vi "play-AFM-CS-imaging_v3.vi"() -> ()   [LabVIEW 2017]
uses:
  controls/boolean_info.ctl
  controls/z-axis-params_v3.ctl
  controls/TF-params.ctl
  <userlib>/_matio/level5/Public/MAT-File Data Types.ctl
  <vilib>/userdefined/High Color/nirio_resource_hc.ctl
  controls/expMetaData.ctl
  <vilib>/Utility/file.llb/Read Delimited Spreadsheet (DBL).vi
  <vilib>/FPGAPlugInAG/cRIO-9082/niLvFpga_Open_cRIO-9082.vi
  <vilib>/rvi/interface/common/dynamic/niFpgaDynamicAddResources.vi
  <vilib>/FPGAPlugInAG/Dynamic/niLvFpga_Reset_Dynamic.vi
  <vilib>/rvi/interface/common/niFpgaWaitOnOcc.vi
  <vilib>/Utility/error.llb/Error Cluster From Error Code.vi
  <vilib>/rvi/errors/niLvFpgaAdjustHostInterfaceError.vi
  <vilib>/FPGAPlugInAG/Dynamic/niLvFpga_Run_Dynamic.vi
  fpga_interface_lib/acquire_FXP_16-5_FIFO_2.vi
  <vilib>/Utility/file.llb/Write Delimited Spreadsheet (DBL).vi
  <vilib>/FPGAPlugInAG/Dynamic/niLvFpga_Close_Dynamic.vi
  <userlib>/_matio/level5/Public/Write/Append Data Element.llb/Append Data Element (Anything).vi
  <vilib>/rvi/interface/nirviOpenFPGA/nirviOpenFPGA.xnode
  FPGA Bitfiles/afmimagingcontro_FPGATargetSPARTA_cs-scanningv3.lvbitx
  <vilib>/rvi/interface/nirviMethod/nirviMethod.xnode
  <vilib>/rvi/interface/nirviReadWriteControl/nirviReadWriteControl.xnode
  <vilib>/rvi/interface/nirviCloseFPGA/nirviCloseFPGA.xnode
  <vilib>/FPGAPlugInAG/Dynamic/niLvFpga_ConfigureFifo_Dynamic.vi
  <vilib>/rvi/errors/niLvFpgaMergeErrorWithErrorCode.vi
  <vilib>/rvi/interface/Simulation/niFpgaSimulationCallBeginRW.vi
  NiFpgaLv.dll
  <userlib>/_matio/level5.lvlib
  fpga_interface_lib/fpga_interface.lvlib
panel:
  in  "do-Dz":bool
  in  "TF-params":T1={"TF-order"=2, "Num"=[1.0237086, -2.0434425, 1.0225973, 0.0, 0.0, 0.0, 0.0, 0.0, 0.0], "Den"=[1.0, -1.9961116, 0.998975, 0.0, 0.0, 0.0, 0.0, 0.0, 0.0]}
  in  "input-data-path":path
  out "boolean \nindicators":T2
  out "CS Time":dbl
  out "Current Case":i16
  out "state times":dbl[](array[numeric])
  out "entity-index":i16
  in  "Tab Control":T3(tab)
  in  "init Z up":sgl step=0.5
  in  "trigger-0":bool
  in  "numEntities":i16
  out "output-data-path":path
  out "output-meta-data-path":path
  in  "note-blob":string
  in  "overwrite":bool
  in  "TsTicks":u32=1600
  in  "Ki-xy":sgl=0.005
  in  "collect all":bool=TRUE
  in  "z_axis_params":T4={"TOL"=0.01, "ramp_rate"=-0.005, "z_u_max"=6.0, "setpoint"=0.0, "Ki"=0.04, "Z_error_threshold"=0.05, "Z_settled_samples_threshold "=500, "zup_rate"=0.1, "uz_safe"=0.60009765625, "Kiz_down"=0.04, "max_Z_settle_samples"=2500} {"uz_safe" format="%#_13g"; "Z_error_threshold" format="%#_13g"; "ramp_rate" format="%#_4g"; "TOL" format="%#_13g"}
  in  "ramp_down":bool
  in  "xy settled-samples\n threshold":i16=200
  in  "xy error-threshold":sgl=0.1
  out "number-settled-samples-x":i16
  out "number-settled-samples-y":i16
  out "case-selected":i16
  out "number-settled-samples-Z":i16
  out "size(s)":i32
  out "nsamps":i32
  out "y iter":i32
  out "size(s) 2":i32[](array[numeric])
  out "Array":i32[][](array[numeric])
  out "error out 2":errorcluster
  out "z-control":dbl[](graph)
  out "x-axis":dbl[](graph)
  out "z-error":dbl[](graph)
  out "y-axis":dbl[](graph)
  in  "STOP":bool
  # "- If collect all = fasle and collect move = false,\nwe only collect measurement data.\n- If collect all = false, and collect move = true,\nwe collect measurement and move data.\n- If collect all = true, we collect everything."
  # "move"
  # "lower"
  # "z-settle"
  # "scan"
  # "tip-up"
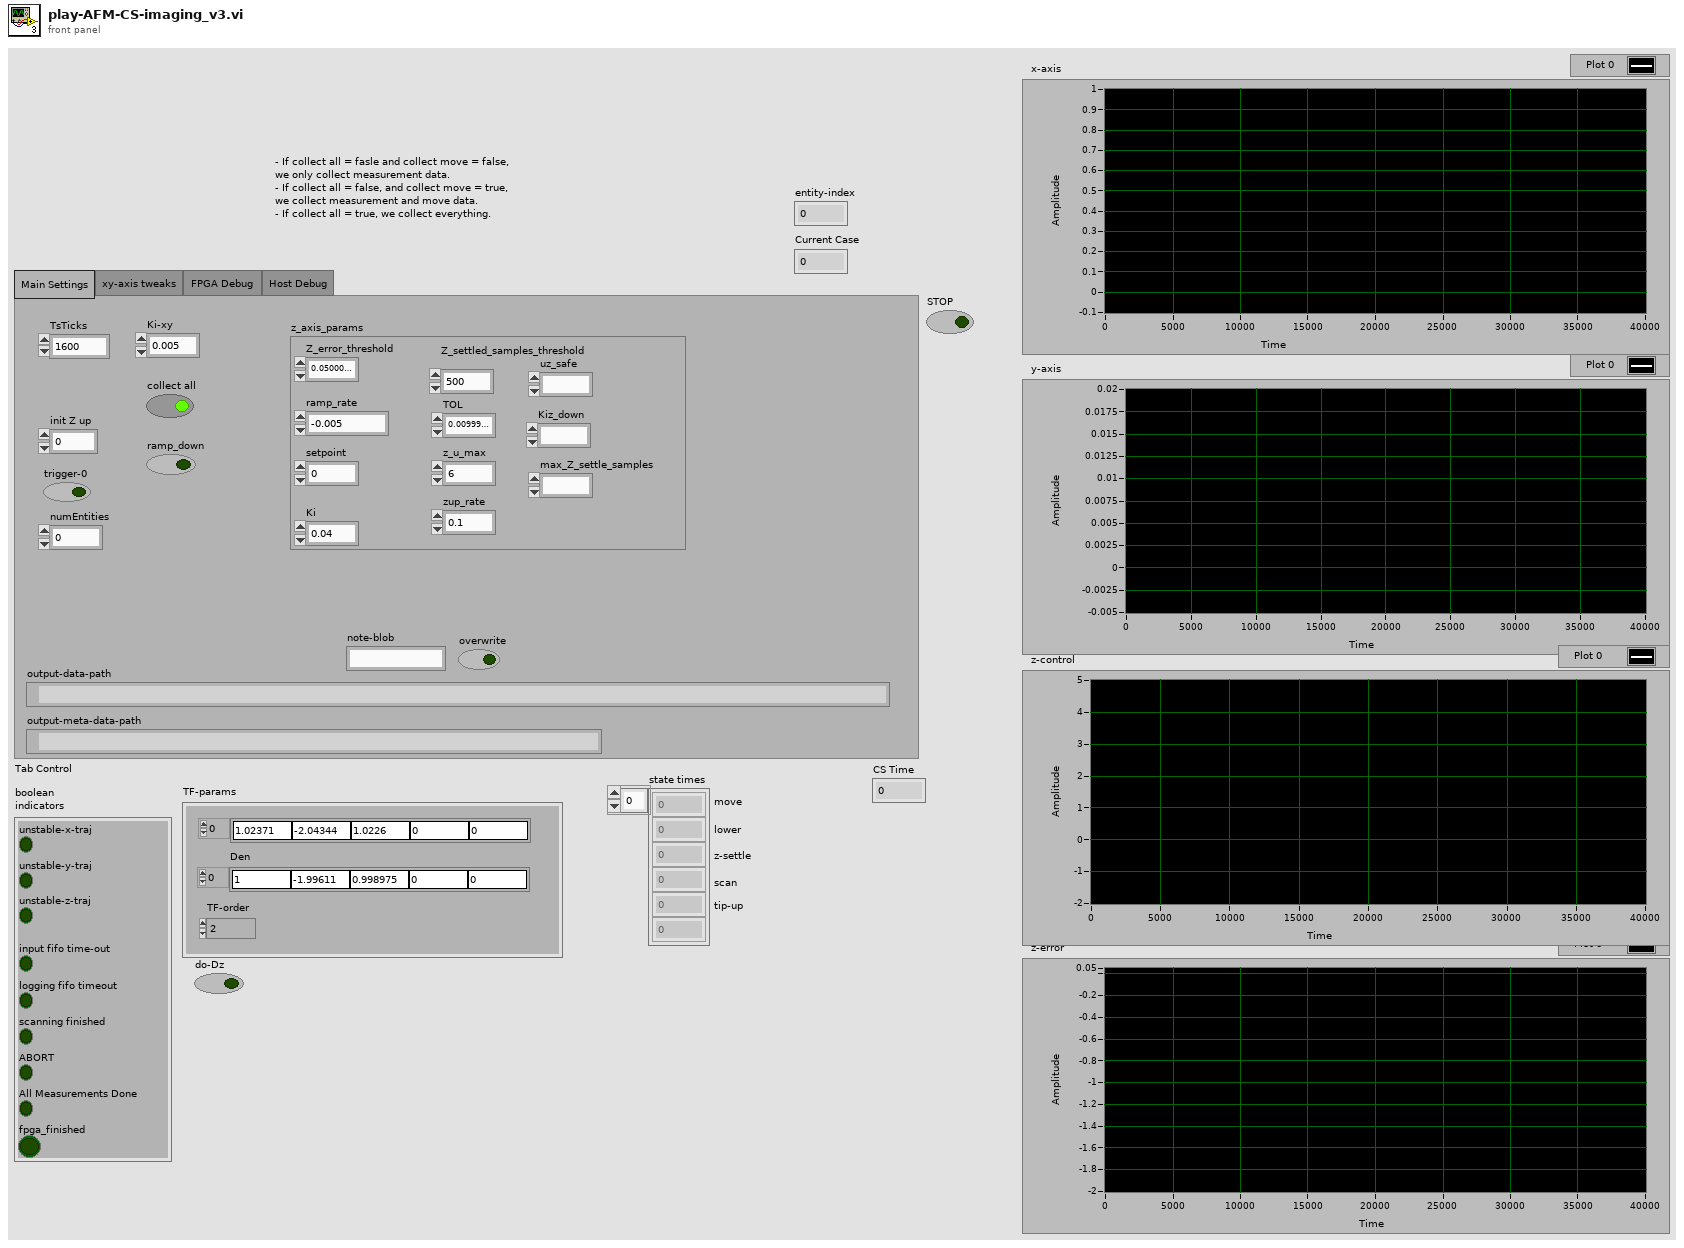
[diagram p1: front panel]
types:
  T1 = typedef "TF-params.ctl" = cluster{"TF-order":i16, "Num":sgl[], "Den":sgl[]}
  T2 = typedef "boolean_info.ctl" = cluster{"unstable-z-traj":bool, "input fifo time-out":bool, "logging fifo timeout":bool, "scanning finished":bool, "unstable-x-traj":bool, "unstable-y-traj":bool, "ABORT":bool, "All Measurements Done":bool, "fpga_finished":bool}
  T3 = enum32{"Main Settings", "xy-axis tweaks", "FPGA Debug ", "Host Debug"}
  T4 = typedef "z-axis-params_v3.ctl" = cluster{"TOL":sgl, "ramp_rate":sgl, "z_u_max":sgl, "setpoint":sgl, "Ki":sgl, "Z_error_threshold":sgl, "Z_settled_samples_threshold ":i16, "zup_rate":sgl, "uz_safe":fxp<+/-,16,5>, "Kiz_down":sgl, "max_Z_settle_samples":i16}
  T5 = typedef "level5.lvlib/MAT-File Data Types.ctl" = enum32{"_invalid", "miINT8", "miUINT8", "miINT16", "miUINT16", "miINT32", "miUINT32", "miSINGLE", "_reserved_1", "miDOUBLE", "_reserved_2", "_reserved_3", "miINT64", "miUINT64", "miMATRIX", "miCOMPRESSED", "miUTF8", "miUTF16", "miUTF32"}
  T6 = typedef "nirio_resource_hc.ctl" = tag
  T7 = cluster{"unstable-z-traj":bool, "input fifo time-out":bool, "logging fifo timeout":bool, "scanning finished":bool, "unstable-x-traj":bool, "unstable-y-traj":bool, "ABORT":bool, "All Measurements Done":bool, "fpga_finished":bool}
  T8 = enum16{"open", "replace", "create", "open or create", "replace or create", "replace or create with confirmation"}
  T9 = typedef "expMetaData.ctl" = cluster{"xy_error_threshold":sgl, "xy_settled_samples_threshold":i16, "Ki_xy":sgl, "state_counts":dbl[], "TOL":sgl, "ramp_rate":sgl, "z_u_max":sgl, "setpoint":sgl, "Ki":sgl, "Z_error_threshold":sgl, "Z_settled_samples_threshold ":i16, "z_UP":sgl, "zup_N":i16, "Num":sgl[], "Den":sgl[], "max_Z_settle_samples":i16, "Kiz_down":sgl, "do_xy_CL":bool, "do_Alt_Ztrigger":bool, "output-data-path":path, "input-data-path":path, "uz_safe":sgl, "zup_rate":sgl}
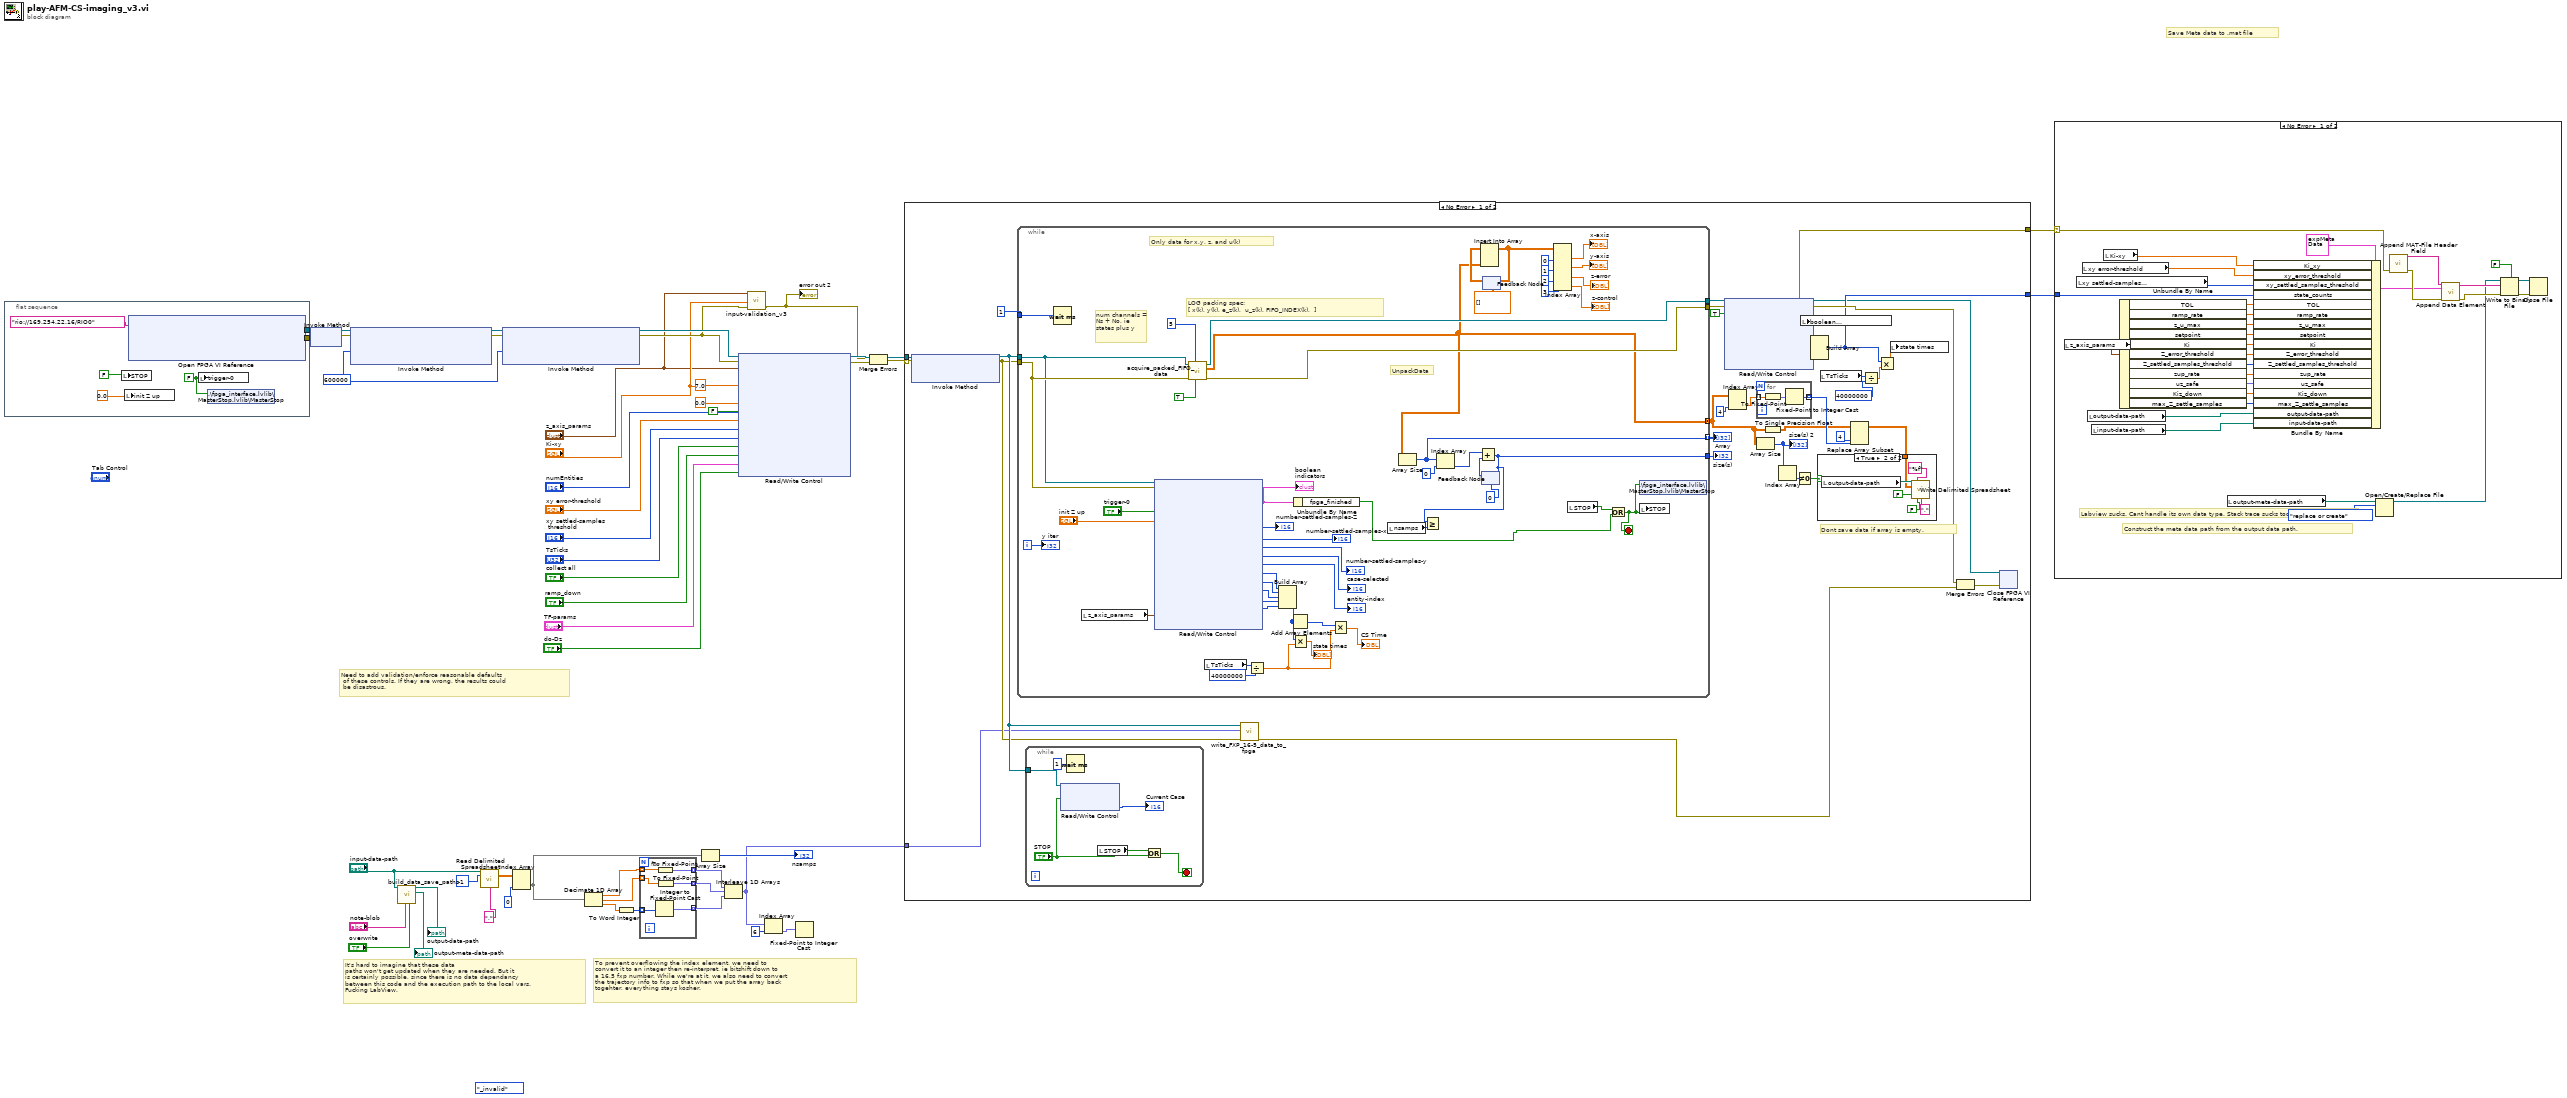
[diagram p0: block diagram]
diagram:
  (unwired) MAT-File_Data_Types."_invalid" ("MAT-File Data Types")
  w48 = 600000
  # "It's hard to imagine that these data\npaths won't get updated when they are needed. But it \nis certainly possible, since there is no data dependancy \nbetween this code and the execution path to the local vars.\nFucking LabView."
  # "Save Meta data to .mat file"
  # "To prevent overflowing the index element, we need to \nconvert it to an integer then re-interpret, ie bitshift down to \na 16,5 fxp number. While we're at it, we also need to convert\nthe trajectory info to fxp so that when we put the array back\ntogehter, everything stays kosher."
  # "Need to add validation/enforce reasonable defaults\n of these controls. If they are wrong, the results could\n be disastrous."
  n1 = flat-sequence {
    tunnel: [w55] -> w47
    tunnel: [w54] -> w46
    frame #0 {
      w50 = FALSE ("trigger-0")
      n2 = local write "STOP"(FALSE) -> ()
      n3 = local write "init Z up"(0.0) -> ()
      n4 = xnode "Open FPGA VI Reference"("resource name"=T6 "rio://169.254.22.16/RIO0") -> ("FPGA VI Reference Out"=w55:refnum<k20>, "error out"=w54:errorcluster)  [unwired: 1 in]
      n5 = local write "trigger-0"(w50) -> ()
      n6 = shared-variable ".\\fpga_interface.lvlib\\MasterStop.lvlib\\MasterStop"(w50) -> ()  [unwired: 1 in, 1 out]
    }
  }
  n7 = xnode "Invoke Method"("FPGA VI Reference In"=w47, "error in"=w46) -> ("FPGA VI Reference Out"=w41:refnum<k20>, "error out"=w40:errorcluster)
  n8 = xnode "Invoke Method"("FPGA VI Reference In"=w41, "error in"=w40, "Requested Depth"=w48) -> ("FPGA VI Reference Out"=w43:refnum<k20>, "error out"=w44:errorcluster)  [unwired: 1 out]
  n9 = call "build_data_save_paths.vi"("overwrite"="overwrite", "note-blob"="note-blob", "input-file"="input-data-path") -> ("output-meta-data-path"=→"output-meta-data-path":path, "output-data-path"=→"output-data-path":path)  [unwired: 5 in, 2 out]
  n10 = call-poly <vilib>:"Read Delimited Spreadsheet.vi"("file path (dialog if empty)"="input-data-path", "number of rows (all:-1)"=-1, "delimiter (\\t)"=",") -> ("all rows"=w36:dbl[][])  [unwired: 7 in, 5 out]
  n11 = xnode "Invoke Method"("FPGA VI Reference In"=w43, "error in"=w44, "Requested Depth"=w48) -> ("FPGA VI Reference Out"=w49:refnum<k20>, "error out"=w8:errorcluster)  [unwired: 1 out]
  n12 = Index Array(array=w36, index (col)=0 ("dimension size")) -> (element=w18:dbl[])  [unwired: 1 in]
  n13 = Decimate 1D Array(w18) -> (w26:dbl[], w25:dbl[], w27:dbl[])
  n14 = To Word Integer(number=w27) -> (16bit integer=w24:i16[])
  n15 = for {
    tunnel: w26 -> [w61] mode=indexing
    tunnel: w25 -> [w60] mode=indexing
    tunnel: [w59] -> w22 mode=indexing
    tunnel: [w58] -> w23 mode=indexing
    tunnel: w24 -> [w57] mode=indexing
    tunnel: [w56] -> w21 mode=indexing
    n16 = Integer to Fixed-Point Cast(integer=w57) -> (fixed-point=w56:fxp<+/-,16,5>)  [unwired: 1 in]
    n17 = To Fixed-Point(number=w61) -> (fixed-point=w58:fxp<+/-,16,5>)  [unwired: 1 in]
    n18 = To Fixed-Point(number=w60) -> (fixed-point=w59:fxp<+/-,16,5>)  [unwired: 1 in]
  }
  n19 = Array Size(array=w18) -> (size(s)=→"nsamps":i32)
  n20 = Interleave 1D Arrays(w23, w22, w21) -> (w17:fxp<+/-,16,5>[])
  n21 = xnode "Read/Write Control"("FPGA VI Reference In"=w49, "error in"=w8, "z_axis_params"="z_axis_params", "xy-bound"=sgl 7.0, "Ki-xy"="Ki-xy", "init Z up"=sgl 0.0 ("u(0)"), "trigger-0"=FALSE, "numEntities"="numEntities", "xy-error-threshold"="xy error-threshold", "settled-samples threshold"="xy settled-samples\n threshold", "TsTicks"="TsTicks", "collect all"="collect all", "ramp_down"="ramp_down", "TF-params"="TF-params", "do-Dz"="do-Dz") -> ("FPGA VI Reference Out"=w42:refnum<k20>, "error out"=w28:errorcluster)
  n22 = call "input-validation_v3.vi"("error constant"=w8, "Ki-xy"="Ki-xy", "z_axis_params"="z_axis_params") -> ("error out"=w7:errorcluster)  [unwired: 8 in]
  "error out 2" <- w7
  n23 = Index Array(array=w17, index=6) -> (element=w20:fxp<+/-,16,5>)
  n24 = Fixed-Point to Integer Cast(1:w20) -> ()  [unwired: 1 out]
  n25 = Merge Errors(w7, w28) -> (w9:errorcluster)
  n26 = case shown="No Error" w9 {
    selector: w9 -> [w66 w164]
    tunnel: w42 -> [w97 _]
    tunnel: w17 -> [w63 _]
    tunnel: [w96 w164] -> w15
    tunnel: [w95 _] -> w14
    frame No Error {
      # "Dont save data if array is empty."
      n27 = xnode "Invoke Method"("FPGA VI Reference In"=w97, "error in"=w66) -> ("FPGA VI Reference Out"=w65:refnum<k20>, "error out"=w64:errorcluster)  [unwired: 1 in]
      n28 = while {
        tunnel: 1 -> [w163]
        tunnel: w65 -> [w118]
        tunnel: w64 -> [w119]
        tunnel: [w116] -> w91
        tunnel: [w114] -> w82 mode=concatenating
        tunnel: [w156] -> w93
        tunnel: [w115] -> w90
        tunnel: [w152] -> w87 mode=indexing
        i -> [w157]
        stop <- w120 stop-if-true
        # "LOG packing spec:\n[ x(k), y(k), e_z(k),  u_z(k), FIFO_INDEX(k),  ]"
        # "num channels = Ns + No, ie states plus y"
        # "Only data for x,y, z, and u(k)"
        # "UnpackData"
        n29 = Wait (ms)(milliseconds to wait=w163) -> ()  [unwired: 1 out]
        n30 = local read "z_axis_params"() -> (w124:T4)
        n31 = xnode "Read/Write Control"("FPGA VI Reference In"=w118, "error in"=w119, "trigger-0"="trigger-0", "init Z up"="init Z up", "z_axis_params"=w124) -> ("boolean  indicators"=w128:T7, "number-settled-samples-Z"=→"number-settled-samples-Z":i16, "number-settled-samples-x"=→"number-settled-samples-x":i16, "number-settled-samples-y"=→"number-settled-samples-y":i16, "Current Case"=→"case-selected":u8, "entity-index"=→"entity-index":i16, "state1-count"=w123:u64, "state2-count"=w122:u64, "state3-count"=w121:u64, "state4-count"=w136:u64, "state5-count"=w135:u64)  [unwired: 1 in, 3 out]
        "boolean \nindicators" <- w128
        n32 = call-poly "acquire_packed_FIFO_data.vi"("Run once?"=TRUE, "numChannels"=u32 5 ("y"), "error in"=w119, "FPGA Interface(in)"=w118) -> ("error out"=w115:errorcluster, "2D Data Out"=w114:dbl[][], "FPGA VI Reference Out"=w116:refnum<k20>)  [unwired: 3 in, 2 out]
        n33 = local read "TsTicks"() -> (w131:u32)
        n34 = Divide(x=w131, y=u32 40000000) -> (x/y=w126:dbl)
        n35 = Build Array(w123, w122, w121, w136, w135) -> (w127:u64[])
        n36 = Add Array Elements(numeric array=w127) -> (sum=w132:u64)
        n37 = Multiply(x=w127, y=w126) -> (x*y=→"state times":dbl[])
        n38 = Unbundle By Name(w128) -> ("fpga_finished"=w138:bool)
        n39 = Multiply(x=w132, y=w126) -> (x*y=→"CS Time":dbl)
        n40 = local read "nsamps"() -> (w161:i32)
        n41 = Array Size(array=w114) -> (size(s)=w152:i32[])
        n42 = Index Array(array=w152, index=0) -> (element=w159:i32)
        n43 = feedback #1(0) -> (w160:i32)
        n44 = Add(x=w159, y=w160) -> (x+y=w156:i32)
        n45 = Greater Or Equal?(x=w156, y=w161) -> ()  [unwired: 1 out]
        n46 = feedback-in #1(w156) -> ()
        n47 = feedback #2(dbl[][] []) -> (w148:dbl[][])
        n48 = Insert Into Array(array=w148, new element=w114) -> (w139:dbl[][])  [unwired: 2 in]
        n49 = feedback-in #2(w139) -> ()
        n50 = Index Array(array=w139, index (col) #1=0 ("disabled index (col)"), index (col) #2=1 ("index (col)"), index (col) #3=2 ("index (col)"), index (col) #4=3 ("index (col)")) -> (element #1=→"x-axis":dbl[], element #2=→"y-axis":dbl[], element #3=→"z-error":dbl[], element #4=→"z-control":dbl[])  [unwired: 4 in]
        n51 = local read "STOP"() -> (w153:bool)
        n52 = Or(x=w153, y=w138) -> (x .or. y?=w120:bool)
        n53 = shared-variable ".\\fpga_interface.lvlib\\MasterStop.lvlib\\MasterStop"(w120) -> ()  [unwired: 1 in, 1 out]
        n54 = local write "STOP"(w120) -> ()
        "y iter" <- w157
      }
      "size(s)" <- w93
      "Array" <- w87
      n55 = while {
        tunnel: w65 -> [w112]
        stop <- w108 stop-if-true
        n56 = xnode "Read/Write Control"("FPGA VI Reference In"=w112, "ABORT"="STOP") -> ("Current Case"=→"Current Case":u8)  [unwired: 1 in, 2 out]
        n57 = Wait (ms)(milliseconds to wait=u32 1) -> ()  [unwired: 1 out]
        n58 = local read "STOP"() -> (w109:bool)
        n59 = Or(x=w109, y="STOP") -> (x .or. y?=w108:bool)
      }
      n60 = call "write_FXP_16-5_data_to_fpga.vi"("error in"=w64, "all rows"=w63, "FPGA Interface"=w65) -> ("error out"=w62:errorcluster)  [unwired: 7 in, 1 out]
      n61 = xnode "Read/Write Control"("FPGA VI Reference In"=w91, "error in"=w90, "ABORT"=TRUE) -> ("FPGA VI Reference Out"=w88:refnum<k20>, "error out"=w96:errorcluster, "boolean  indicators"=w71:T7, "state1-count"=w80:u64, "state2-count"=w79:u64, "state3-count"=w78:u64, "state4-count"=w77:u64, "state5-count"=w76:u64)
      n62 = Index Array(array=w82, index (col)=4) -> (element=w85:dbl[])  [unwired: 1 in]
      n63 = for {
        tunnel: w85 -> [w105] mode=indexing
        tunnel: [w106] -> w83 mode=indexing
        n64 = To Fixed-Point(number=w105) -> (fixed-point=w104:fxp<+/-,16,5>)  [unwired: 1 in]
        n65 = Fixed-Point to Integer Cast(1:w104) -> (0:w106:i16)
      }
      n66 = Array Size(array=w82) -> (size(s)=w72:i32[])
      "size(s) 2" <- w72
      n67 = To Single Precision Float(number=w82) -> (single precision float=w81:sgl[][])
      n68 = Index Array(array=w72) -> (element=w73:i32)  [unwired: 1 in]
      n69 = Not Equal To 0?(x=w73) -> (x != 0?=w74:bool)
      n70 = local write "boolean \nindicators"(w71) -> ()
      n71 = Build Array(w80, w79, w78, w77, w76) -> (w95:u64[])
      n72 = local read "TsTicks"() -> (w70:u32)
      n73 = Replace Array Subset(array=w81, new element=w83, index (col)=4) -> (w75:sgl[][])  [unwired: 1 in]
      n74 = case shown="True" w74 {
        tunnel: w75 -> [_ w98]
        frame False {
        }
        frame True {
          n75 = local read "output-data-path"() -> (w103:path)
          n76 = call-poly <vilib>:"Write Delimited Spreadsheet.vi"("file path (dialog if empty)"=w103, "format (%.3f)"="%f", "2D data"=w98, "append to file? (new file:F)"=FALSE, "transpose? (no:F)"=FALSE, "delimiter (\\t)"=",") -> ()  [unwired: 8 in, 2 out]
        }
      }
      n77 = Divide(x=w70, y=u32 40000000) -> (x/y=w68:dbl)
      n78 = Multiply(x=w95, y=w68) -> (x*y=w67:dbl[])
      n79 = local write "state times"(w67) -> ()
      n80 = Merge Errors(w96, w62) -> (w92:errorcluster)
      n81 = xnode "Close FPGA VI Reference"("FPGA VI Reference In"=w88, "error in"=w92) -> ()  [unwired: 1 out]
    }
    frame Error {
    }
  }
  n82 = case shown="No Error" w15 {
    selector: w15 -> [w188 _]
    tunnel: w14 -> [w177 _]
    frame No Error {
      # "Construct the meta data path from the output data path."
      # "Labview sucks. Cant handle its own data type. Stack trace sucks too."
      n83 = local read "z_axis_params"() -> (w176:T4)
      n84 = local read "xy settled-samples\n threshold"() -> (w173:i16)
      n85 = local read "xy error-threshold"() -> (w174:sgl)
      n86 = local read "output-data-path"() -> (w166:path)
      n87 = local read "input-data-path"() -> (w167:path)
      n88 = local read "Ki-xy"() -> (w175:sgl)
      n89 = Unbundle By Name(w176) -> ("TOL"=w185:sgl, "ramp_rate"=w184:sgl, "z_u_max"=w183:sgl, "setpoint"=w182:sgl, "Ki"=w181:sgl, "Z_error_threshold"=w180:sgl, "Z_settled_samples_threshold"=w179:i16, "zup_rate"=w170:sgl, "uz_safe"=w169:fxp<+/-,16,5>, "Kiz_down"=w168:sgl, "max_Z_settle_samples"=w165:i16)
      n90 = local read "output-meta-data-path"() -> (w171:path)
      n91 = Bundle By Name(cluster=T9 {"xy_error_threshold"=0.1, "xy_settled_samples_threshold"=200, "Ki_xy"=0.005, "state_counts"=[], "TOL"=0.3, "ramp_rate"=-5e-06, "z_u_max"=5.0, "setpoint"=0.0, "Ki"=0.001, "Z_error_threshold"=0.0, "Z_settled_samples_threshold "=0, "z_UP"=1.5, "zup_N"=5000, "Num"=[-0.00254, 0.000408, 0.00295, 0.0, 0.0, 0.0, 0.0, 0.0, 0.0], "Den"=[0.982758, -1.98194, 1.0, 0.0, 0.0, 0.0, 0.0, 0.0, 0.0], "max_Z_settle_samples"=5000, "Kiz_down"=0.001, "do_xy_CL"=FALSE, "do_Alt_Ztrigger"=FALSE, "output-data-path"=path "", "input-data-path"=path "", "uz_safe"=0.0, "zup_rate"=0.0} ("ExpMetaData"), "Ki_xy"=w175, "xy_error_threshold"=w174, "xy_settled_samples_threshold"=w173, "state_counts"=w177, "TOL"=w185, "ramp_rate"=w184, "z_u_max"=w183, "setpoint"=w182, "Ki"=w181, "Z_error_threshold"=w180, "Z_settled_samples_threshold"=w179, "zup_rate"=w170, "uz_safe"=w169, "Kiz_down"=w168, "max_Z_settle_samples"=w165, "output-data-path"=w166, "input-data-path"=w167) -> (w186:T9)
      n92 = Open/Create/Replace File(file path (use dialog)=w171, operation (0:open)=T8."replace or create") -> (refnum out=w187:refnum<file>)  [unwired: 4 in, 2 out]
      n93 = call <userlib>:"Append MAT-File Header Field.vi"("error"=w188) -> ("result string"=w195:string, "error out"=w189:errorcluster)  [unwired: 13 in]
      n94 = call-poly <userlib>:"Append Data Element.vi"("initial string"=w195, "data"=w186, "error in (no error)"=w189) -> ("result string"=w193:string, "error out"=w194:errorcluster)  [unwired: 11 in]
      n95 = Write to Binary File(file (use dialog)=w187, data=w193, error in=w194, 5:FALSE ("prepend array or string size? (T)")) -> (refnum out=w190:refnum<file>, error out=w191:errorcluster)  [unwired: 2 in, 1 out]
      n96 = Close File(refnum=w190, error in=w191) -> ()  [unwired: 2 out]
    }
    frame Error {
    }
  }
